vi "VHDI-recieveData.vi"(8 "error in (no error)":errorcluster, 10 "Data":T1, 11 "VG-VNA_GUI in":refnum<class "VG-VNA_GUI.lvclass">) -> (0 "error out":errorcluster, 3 "VG-VNA_GUI out":refnum<class "VG-VNA_GUI.lvclass">)   [LabVIEW 2020, in "VG-VNA_GUI.lvlib" / "VG-VNA_GUI.lvclass"]
uses:
  VG-VNA_GUI.lvclass
  data_handler/VDH-VNA_data_handler/VDH-VNA_data_handler/VDH-VNA_data.ctl
  VG-VNA_GUI.lvclass/VG-VNA_GUI.ctl
  data_handler/VDH-VNA_data_handler/VDH-VNA_data_handler/VDH-VNA_data_handler.lvclass
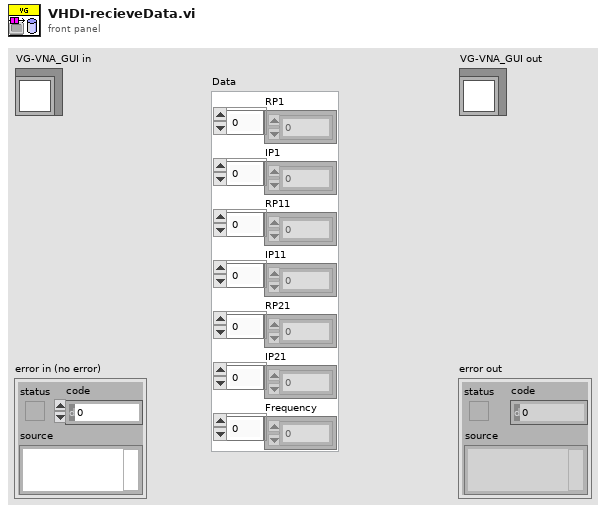
[diagram p1: front panel]
types:
  T1 = typedef "VDH-VNA_data_handler.lvlib/VDH-VNA_data_handler.lvclass/VDH-VNA_data.ctl" = cluster{"RP1":dbl[], "IP1":dbl[], "RP11":dbl[], "IP11":dbl[], "RP21":dbl[], "IP21":dbl[], "Frequency":u64[]}
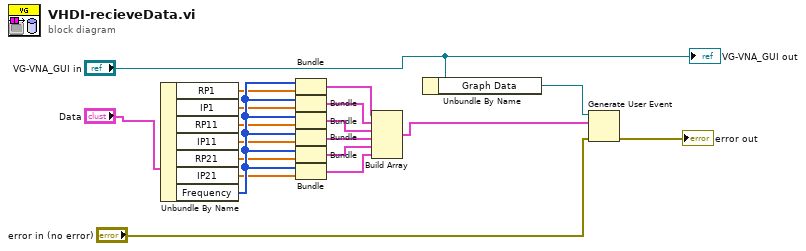
[diagram p0: block diagram]
diagram:
  n1 = Unbundle By Name("Data") -> ("RP1"=w11:dbl[], "IP1"=w10:dbl[], "RP11"=w9:dbl[], "IP11"=w8:dbl[], "RP21"=w7:dbl[], "IP21"=w6:dbl[], "Frequency"=w19:u64[])
  n2 = Bundle("Frequency"=w19, "RP1"=w11) -> (w18:cluster{"Frequency":u64[], "RP1":dbl[]})  [unwired: 1 in]
  n3 = Bundle("Frequency"=w19, "IP1"=w10) -> (w17:cluster{"Frequency":u64[], "IP1":dbl[]})  [unwired: 1 in]
  n4 = Bundle("Frequency"=w19, "RP11"=w9) -> (w14:cluster{"Frequency":u64[], "RP11":dbl[]})  [unwired: 1 in]
  n5 = Bundle("Frequency"=w19, "IP11"=w8) -> (w13:cluster{"Frequency":u64[], "IP11":dbl[]})  [unwired: 1 in]
  n6 = Bundle("Frequency"=w19, "RP21"=w7) -> (w15:cluster{"Frequency":u64[], "RP21":dbl[]})  [unwired: 1 in]
  n7 = Bundle("Frequency"=w19, "IP21"=w6) -> (w16:cluster{"Frequency":u64[], "IP21":dbl[]})  [unwired: 1 in]
  n8 = Build Array(w18, w17, w14, w13, w15, w16) -> (w3:cluster{"Frequency":u64[], "IP21":dbl[]}[])
  n9 = Unbundle By Name("VG-VNA_GUI in") -> ("Graph Data"=w4:refnum<user-event>)
  n10 = Generate User Event(user event=w4, event data cluster=w3, error in="error in (no error)") -> (error out=→"error out":errorcluster)  [unwired: 1 in, 1 out]
  "VG-VNA_GUI out" <- "VG-VNA_GUI in"
